vi "Test SubVI to Code 1.vi"() -> ()   [LabVIEW 2018]
panel:
  out "2nd SubVI C call":string="singal_out_2_wire = Basic_Function_Generator(wireUID_266, wireUID_447);"
  out "1st SubVI C call":string="singal_out_wire = Basic_Function_Generator(ampliltudeWire, frequencyWire);"
  in  "vi path":path=path "C:/Users/lubo/Documents/LabView/LabVIEW-Universal-Transcriptor/Test/Examples For Parsing/Example While Loop Some Operations 1.vi"
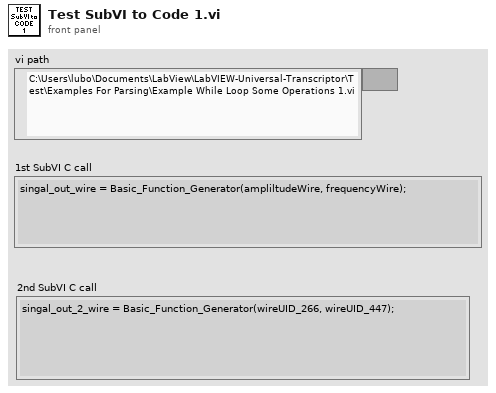
[diagram p1: front panel]
types:
  T1 = cluster{"terminals datatypes":string[][], "terminal\nconnected?":bool[], "terminal captions":string[], "term. count":i32, "terminal\nIsSource?":bool[], "SubVI name":string, "connected\nwires refs.":refnum<vi>[], "coerced\ndot?":bool[], "terminals[]":refnum<vi>[]}
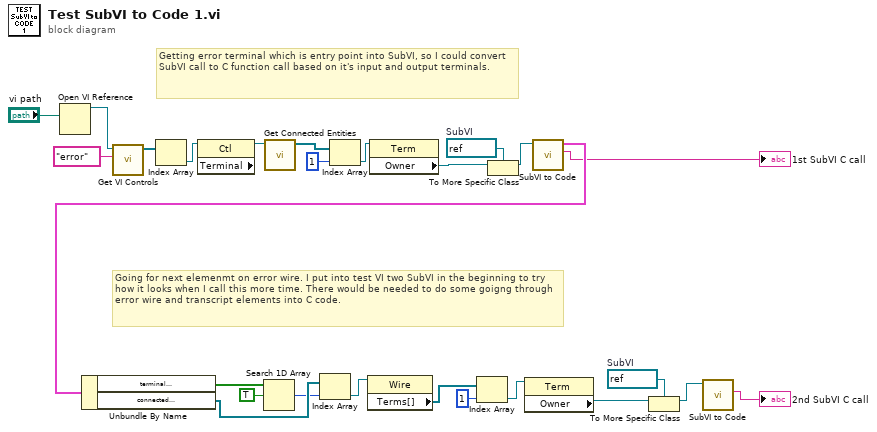
[diagram p0: block diagram]
diagram:
  w5 = refnum<vi> refnum  # SubVI
  w17 = refnum<vi> refnum  # SubVI
  # "Going for next elemenmt on error wire. I put into test VI two SubVI in the beginning to try how it looks when I call this more time. There would be needed to do some goigng through error wire and transcript elements into C code."
  # "Getting error terminal which is entry point into SubVI, so I could convert SubVI call to C function call based on it's input and output terminals."
  n1 = Open VI Reference(vi path="vi path") -> (vi reference=w24:refnum<vi>)  [unwired: 5 in, 1 out]
  n2 = call "Get VI Controls.vi"("DataType"="error", "VI ref."=w24) -> ("Controls Array"=w23:refnum<vi>[])  [unwired: 8 in, 1 out]
  n3 = Index Array(array=w23) -> (element=w22:refnum<vi>)  [unwired: 1 in]
  n4 = property class="Ctl"(reference=w22) -> ("Terminal"=w21:refnum<vi>)  [unwired: 1 in, 2 out]
  n5 = call "Get Connected Entities.vi"("terminal ref."=w21) -> ("Connected Wire.Terminals[]"=w19:refnum<vi>[])  [unwired: 9 in, 1 out]
  n6 = Index Array(array=w19, index=1) -> (element=w18:refnum<vi>)
  n7 = property class="Term"(reference=w18) -> ("Owner"=w16:refnum<vi>)  [unwired: 1 in, 2 out]
  n8 = To More Specific Class(target class=w17, reference=w16) -> (specific class reference=w15:refnum<vi>)  [unwired: 1 in, 1 out]
  n9 = call "SubVI to Code.vi"("reference"=w15) -> ("C code"=→"1st SubVI C call":string, "SubVI terminals info"=w14:T1)  [unwired: 9 in]
  n10 = Unbundle By Name(w14) -> ("terminal\nIsSource?"=w13:bool[], "connected\nwires refs."=w11:refnum<vi>[])
  n11 = Search 1D Array(1D array=w13, element=TRUE) -> (index of element=w10:i32)  [unwired: 1 in]
  n12 = Index Array(array=w11, index=w10) -> (element=w9:refnum<vi>)
  n13 = property class="Wire"(reference=w9) -> ("Terms[]"=w8:refnum<vi>[])  [unwired: 1 in, 2 out]
  n14 = Index Array(array=w8, index=1) -> (element=w6:refnum<vi>)
  n15 = property class="Term"(reference=w6) -> ("Owner"=w4:refnum<vi>)  [unwired: 1 in, 2 out]
  n16 = To More Specific Class(target class=w5, reference=w4) -> (specific class reference=w3:refnum<vi>)  [unwired: 1 in, 1 out]
  n17 = call "SubVI to Code.vi"("reference"=w3) -> ("C code"=→"2nd SubVI C call":string)  [unwired: 9 in, 1 out]
